vi "start.vi"(8 "error in (no error)":errorcluster, 11 "SoundAO in":refnum<class "SoundAO.lvclass">) -> (0 "error out":errorcluster, 3 "SoundAO out":refnum<class "SoundAO.lvclass">)   [LabVIEW 2011, in "Hardware.lvlib" / "Channels.lvlib" / "SoundAO.lvclass"]
doc: "Abstract Method\n\nStarts/Arms the AnalogOutput task. Normally the AnalogOutput device is configured to wait for a trigger signal, therefore, in this case the method Arms the device ready for recieving its trigger upon which it will start outputing immediately its data."
uses:
  SoundAO.lvclass
  SoundAO.lvclass/SoundAO.ctl
  Program Files/National Instruments/LabVIEW 2011/resource/lvsound2.dll
  AnalogOutput.lvclass
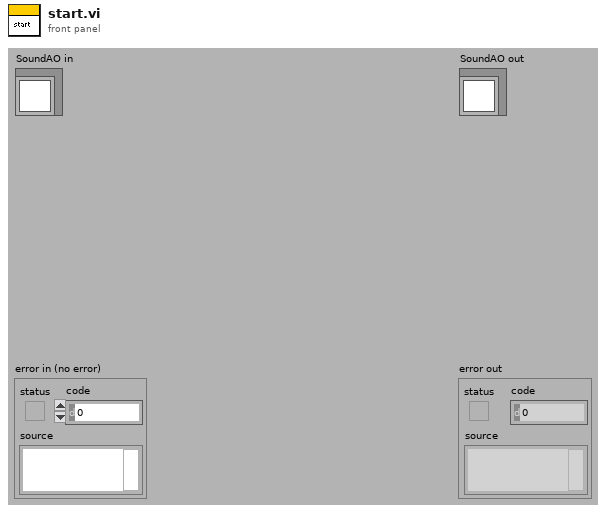
[diagram p1: front panel]
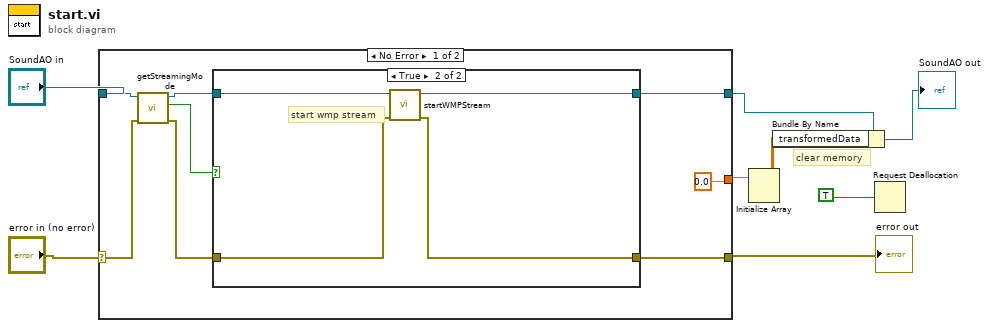
[diagram p0: block diagram]
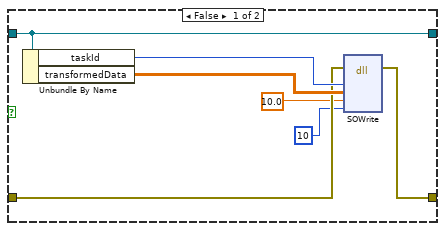
[diagram p2: hidden frame]
diagram:
  # "clear memory"
  n1 = case shown="No Error" "error in (no error)" {
    selector: "error in (no error)" -> [w10 w28]
    tunnel: [w15 w28] -> w7
    tunnel: [w14 w29] -> w4
    tunnel: "SoundAO in" -> [w13 w29]
    tunnel: [0.0 _] -> w2
    frame No Error {
      n2 = call "getStreamingMode.vi"("error in (no error)"=w10, "AnalogOutput.lvclass in"=w13) -> ("error out"=w9:errorcluster, "streamingMode"=w11:bool, "AnalogOutput.lvclass out"=w12:refnum<class "SoundAO.lvclass">)  [unwired: 7 in]
      n3 = case shown="True" w11 {
        tunnel: w12 -> [w17 w27]
        tunnel: w9 -> [w21 w25]
        tunnel: [w20 w24] -> w15
        tunnel: [w17 w26] -> w14
        frame False {
          n4 = Unbundle By Name(w17) -> ("taskId"=w23:i32, "transformedData"=w22:dbl[][])
          n5 = dll-call lib="C:/Program Files/National Instruments/LabVIEW 2011/resource/lvsound2.*" fn="SOWrite"(error in=w21, "taskID"=w23, "DBL Y"=w22, "timeout"=10.0 ("timeout (sec)"), "typeCode"=i16 10) -> (error out=w20:errorcluster)  [unwired: 7 in, 1 out]
        }
        frame True {
          # "start wmp stream"
          n6 = call "startWMPStream.vi"("error in (no error)"=w25, "SoundAO in"=w27) -> ("error out"=w24:errorcluster, "SoundAO out"=w26:refnum<class "SoundAO.lvclass">)  [unwired: 8 in]
        }
      }
    }
    frame Error {
    }
  }
  "error out" <- w7
  n7 = Initialize Array(w2) -> (w3:dbl[][])  [unwired: 2 in]
  n8 = Bundle By Name(cluster=w4, "transformedData"=w3) -> (→"SoundAO out":refnum<class "SoundAO.lvclass">)
  n9 = Request Deallocation(TRUE) -> ()
